vi "Get Configuration.vi"(8 "error in (no error)":errorcluster, 11 "UDP Transfer Tx Configuration in":refnum<class "UDP Transfer Tx Configuration.lvclass">) -> (0 "error out":errorcluster, 2 "transfer settings":T1, 3 "UDP Transfer Tx Configuration out":refnum<class "UDP Transfer Tx Configuration.lvclass">)   [LabVIEW 2017, in "UDP.lvlib" / "UDP Transfer Tx Configuration.lvclass"]
uses:
  UDP Transfer Tx Configuration.lvclass
  Tx Transfer Settings.ctl
  UDP Transfer Tx Configuration.lvclass/UDP Transfer Tx Configuration.ctl
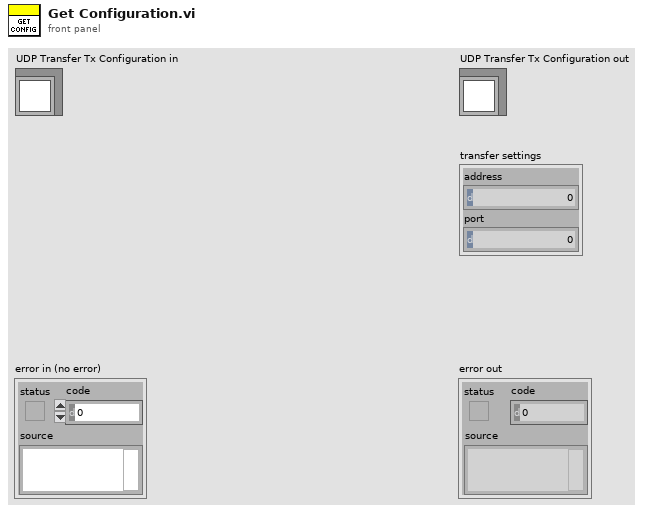
[diagram p1: front panel]
types:
  T1 = typedef "UDP.lvlib/UDP Transfer Tx Configuration.lvclass/Tx Transfer Settings.ctl" = cluster{"address":u32, "port":u16}
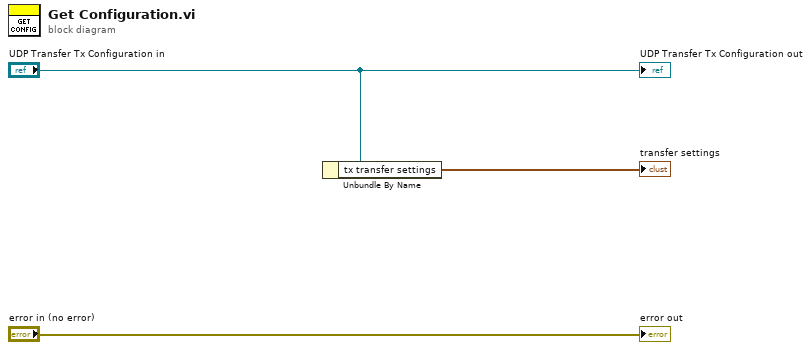
[diagram p0: block diagram]
diagram:
  n1 = Unbundle By Name("UDP Transfer Tx Configuration in") -> ("tx transfer settings"=→"transfer settings":T1)
  "error out" <- "error in (no error)"
  "UDP Transfer Tx Configuration out" <- "UDP Transfer Tx Configuration in"
